vi "Get-processing.vi"(8 "error in (no error)":errorcluster, 11 "Data ref. in":refnum<data-value>) -> (0 "error out":errorcluster, 2 "Processing?":bool, 3 "Data ref.":refnum<data-value>)   [LabVIEW 2013, in "CameraVision.lvlib" / "CV-Main.lvclass"]
uses:
  CV-Main.lvclass
  CV-Main.lvclass/CV-Main.ctl
  Read Processing.vi
  UI/CV-UI.lvclass
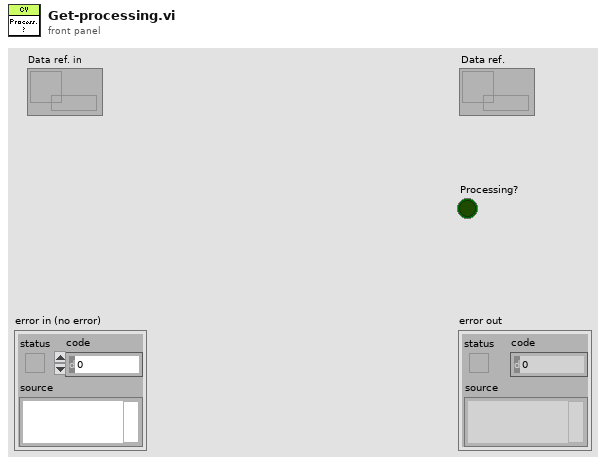
[diagram p1: front panel]
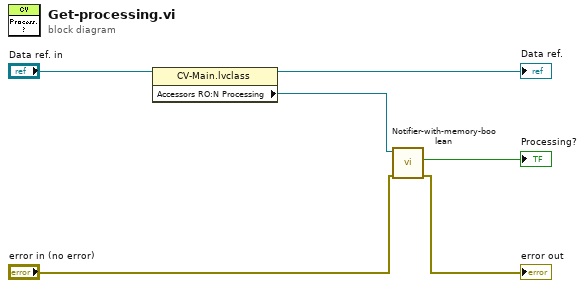
[diagram p0: block diagram]
diagram:
  n1 = property class="CV-Main.lvclass"(reference="Data ref. in") -> (reference out=→"Data ref.":refnum<data-value>, "Accessors RO:N Processing"=w2:refnum<notifier>)  [unwired: 1 in, 1 out]
  n2 = call "Notifier-with-memory-boolean.vi"("error in"="error in (no error)", "Notifier in"=w2) -> ("error IO"=→"error out":errorcluster, "Notification"=→"Processing?":bool)  [unwired: 8 in]
